vi "Teleop - Limit Motion (SubVI).vi"(7 "Desired cluster In":T1 {"shooterMotorMode" items=["PercentOutput"=0, "Position"=1, "Velocity"=2, "Current"=3, "Follower"=5, "MotionProfile"=6, "MotionMagic"=7, "MotionProfileArc"=10, "Disabled"=15]}) -> (8 "Desired cluster Out":T1 {"shooterMotorMode" items=["PercentOutput"=0, "Position"=1, "Velocity"=2, "Current"=3, "Follower"=5, "MotionProfile"=6, "MotionMagic"=7, "MotionProfileArc"=10, "Disabled"=15]})   [LabVIEW 2019]
uses:
  Desired Cluster.ctl
  <vilib>/Rock Robotics/WPI/ThirdParty/Phoenix-LabVIEW/Motor Controller/Controls/CTRE_Phoenix_MotorControl_ControlMode.ctl
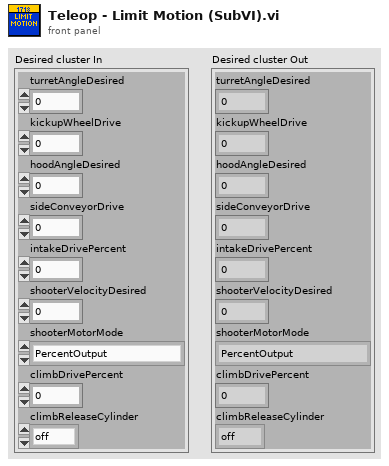
[diagram p1: front panel]
types:
  T1 = typedef "Desired Cluster.ctl" = cluster{"turretAngleDesired":dbl, "kickupWheelDrive":dbl, "hoodAngleDesired":dbl, "sideConveyorDrive":dbl, "intakeDrivePercent":dbl, "shooterVelocityDesired":dbl, "shooterMotorMode":T2, "climbDrivePercent":dbl, "climbReleaseCylinder":enum16{"off", "on", "forward", "back"}}
  T2 = typedef "CTRE_Phoenix_MotorControl_ControlMode.ctl" = u16
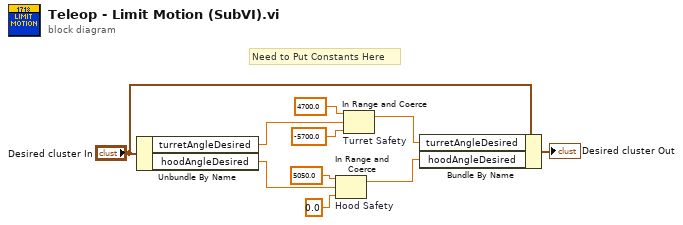
[diagram p0: block diagram]
diagram:
  # "Need to Put Constants Here"
  n1 = Unbundle By Name("Desired cluster In") -> ("turretAngleDesired"=w6:dbl, "hoodAngleDesired"=w5:dbl)
  n2 = In Range and Coerce "Hood Safety"(upper limit=5050.0, x=w5, lower limit=0.0) -> (coerced(x)=w1:dbl)  [unwired: 1 out]
  n3 = In Range and Coerce "Turret Safety"(upper limit=4700.0, x=w6, lower limit=-5700.0) -> (coerced(x)=w2:dbl)  [unwired: 1 out]
  n4 = Bundle By Name(cluster="Desired cluster In", "turretAngleDesired"=w2, "hoodAngleDesired"=w1) -> (→"Desired cluster Out":T1)
